vi "ROS_Status_Publisher_1.vi"() -> ()   [LabVIEW 2016]
uses:
  <userlib>/ROS for LabVIEW Software/ROS/Code/Console/Servers/ServerSubs/TopicDef.ctl
  <userlib>/ROS for LabVIEW Software/ROS/Code/SubVIs/_ROSDirection.ctl
  GlobalVI.vi
  <userlib>/ROS for LabVIEW Software/ROS/MessageBuilding/std_msgs/subs/stringScalar.vi
  <userlib>/ROS for LabVIEW Software/ROS/MessageBuilding/std_msgs/subs/float32Scalar.vi
  <userlib>/ROS for LabVIEW Software/ROS/MessageBuilding/std_msgs/subs/i32Scalar.vi
panel:
  out "JSON string 2":string
  out "error out":errorcluster
  out "UWB_error out":errorcluster
  out "JSON string":string
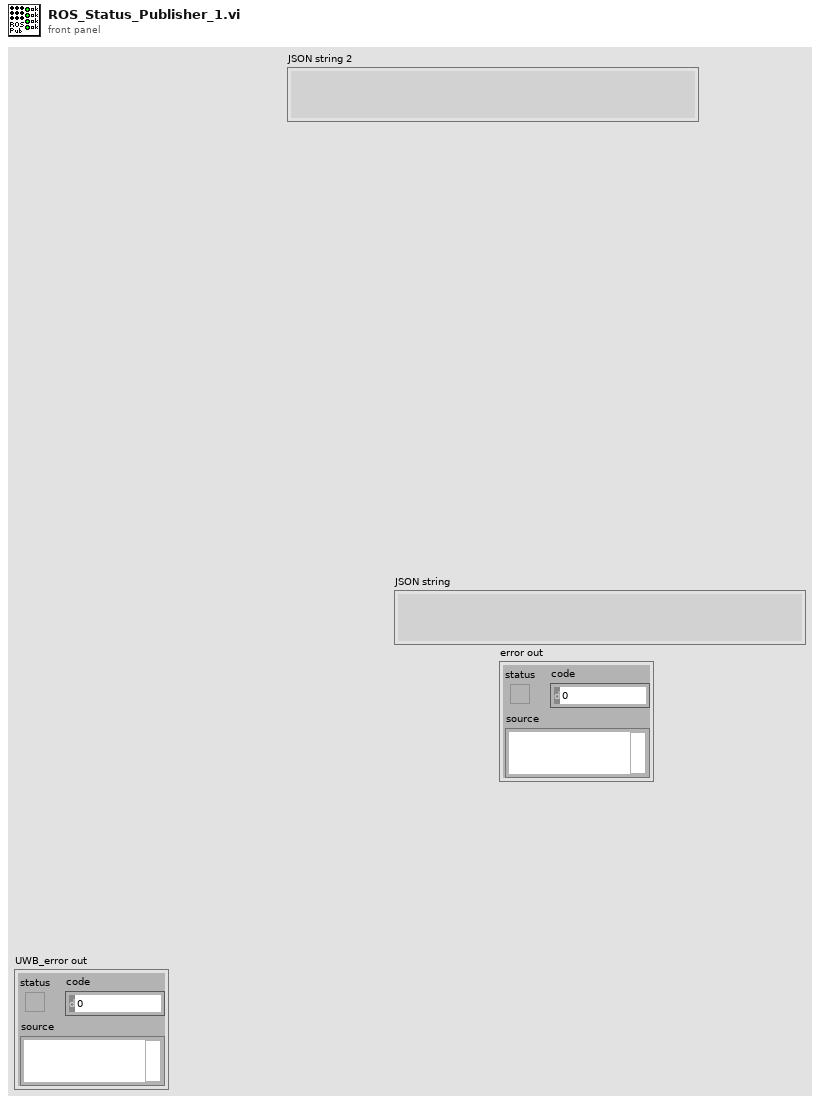
[diagram p1: front panel]
types:
  T1 = typedef "TopicDef.ctl" = cluster{"Topic":string, "Type":string, "Action":T2, "Update (ms)":u16, "queue size":u16}
  T2 = typedef "_ROSDirection.ctl" = enum16{"Node", "Publisher", "Subscriber", "ServiceClient", "ServiceProvider"}
  T3 = cluster{"status":cluster{"liftStatus":bool, "lidarBackStatus":bool, "uwbStatus":bool, "lightStatus":bool}}
  T4 = typedef "_ROSControl.ctl" = cluster{"topic port":u16, "Node":string, "topic":string, "type":string, "node port":u16, "error ":errorcluster, "Direction":T2, "Update (ms)":u16, "FIFO size":u16}
  T5 = cluster{"liftStatus":bool, "lidarBackStatus":bool, "uwbStatus":bool, "lightStatus":bool}
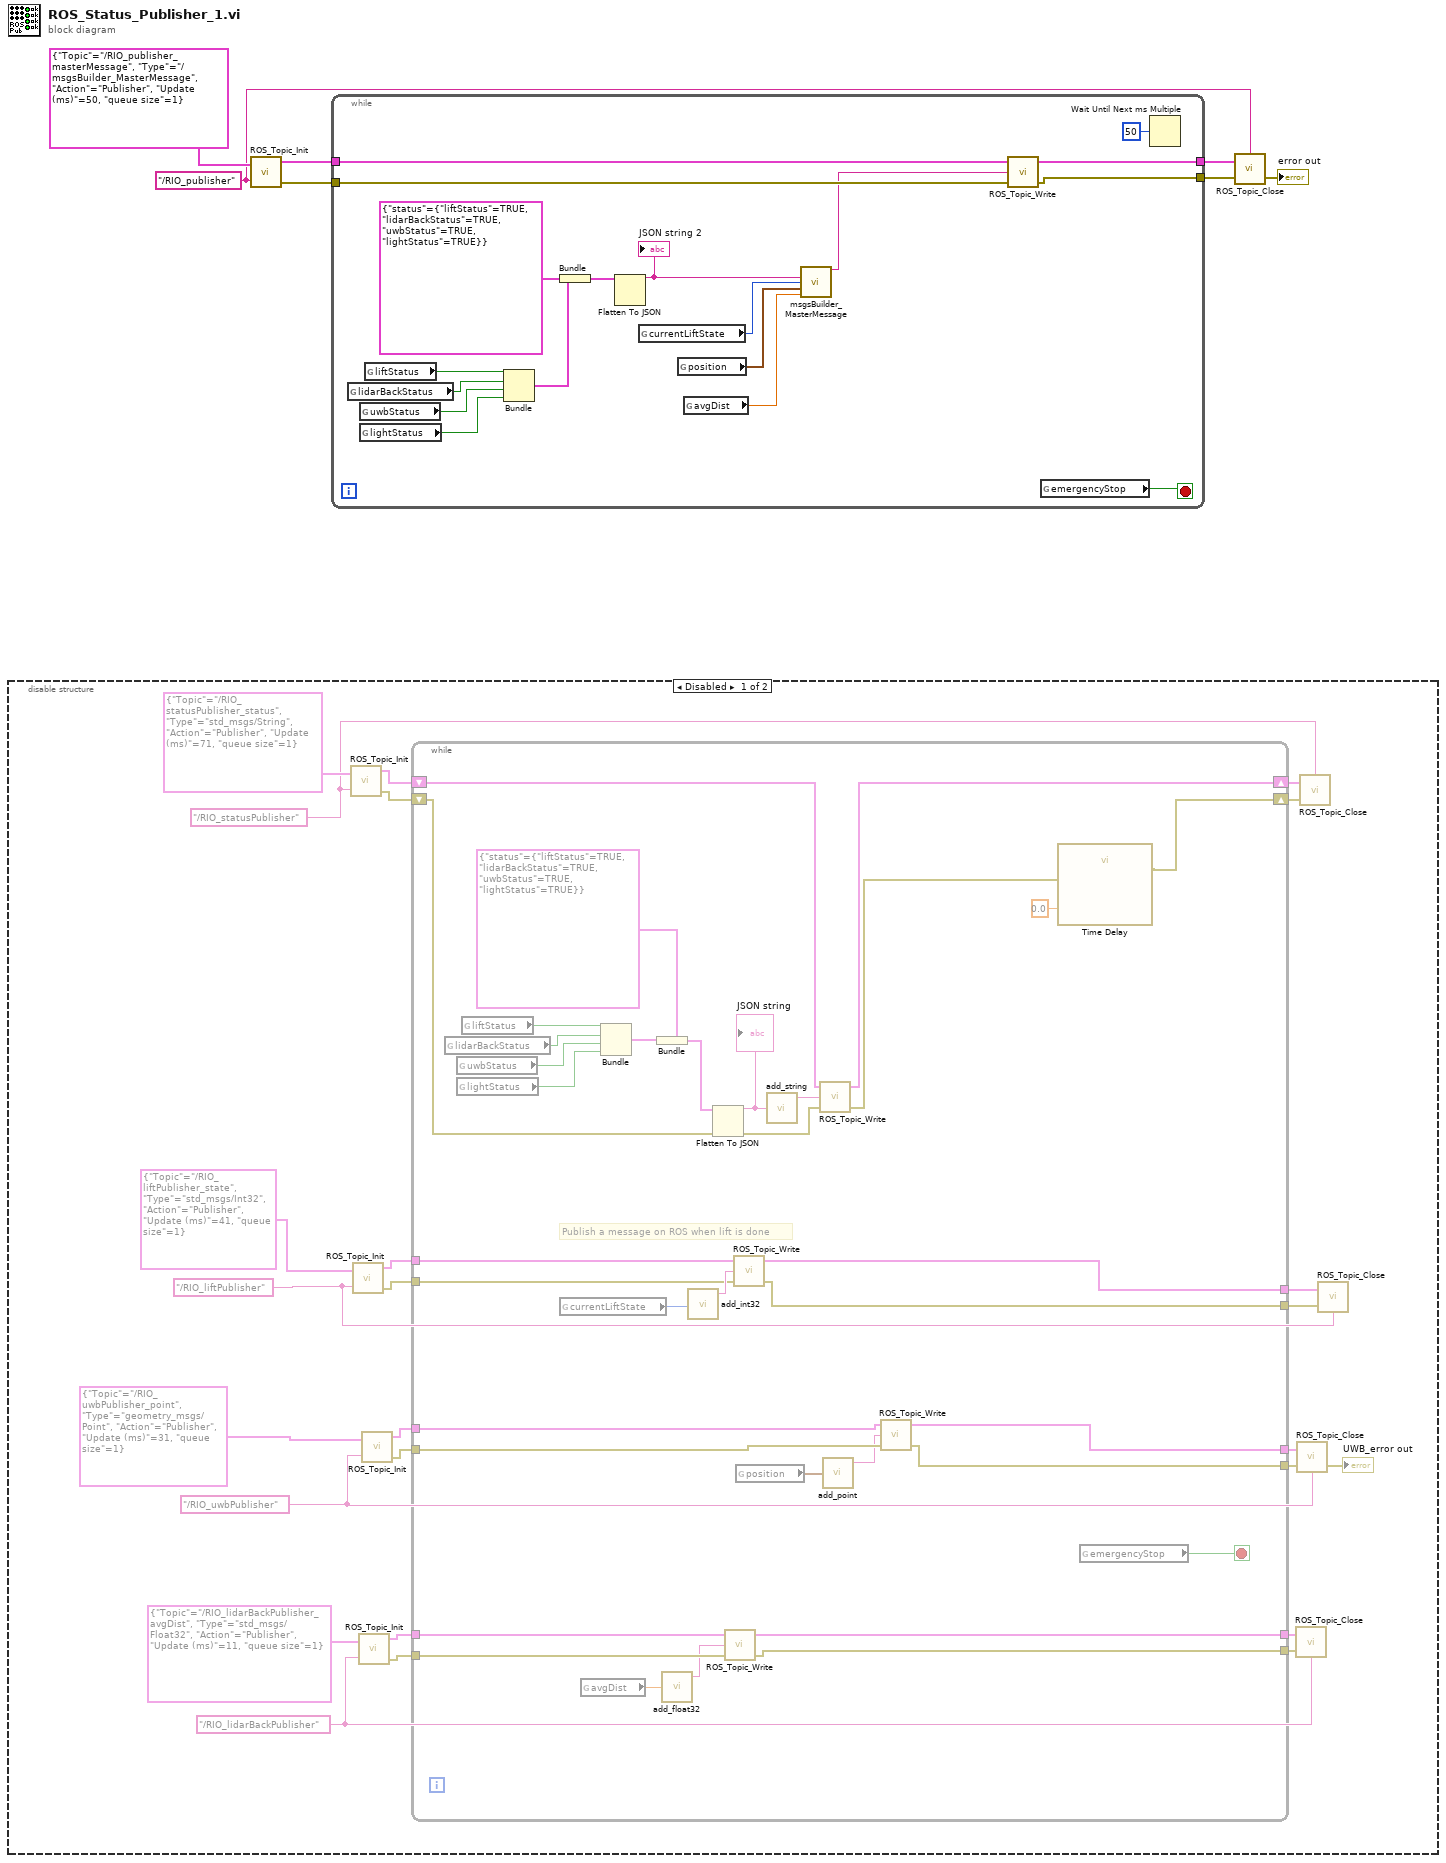
[diagram p0: block diagram]
diagram:
  w6 = "/RIO_publisher" ("node")
  n1 = disable-structure shown="Disabled" {
    frame Disabled {
      w12 = "/RIO_lidarBackPublisher" ("node")
      w14 = "/RIO_liftPublisher" ("node")
      w15 = "/RIO_uwbPublisher" ("node")
      w27 = "/RIO_statusPublisher" ("node")
      n2 = call <userlib>:"ROS_Topic_Init.vi"("Definitions"=T1 {"Topic"="/RIO_statusPublisher_status", "Type"="std_msgs/String", "Action"=enum."Publisher", "Update (ms)"=71, "queue size"=1}, "node"=w27) -> ("ROS out"=w31:T4, "error out"=w29:errorcluster)  [unwired: 1 in]
      n3 = call <userlib>:"ROS_Topic_Init.vi"("Definitions"=T1 {"Topic"="/RIO_liftPublisher_state", "Type"="std_msgs/Int32", "Action"=enum."Publisher", "Update (ms)"=41, "queue size"=1}, "node"=w14) -> ("ROS out"=w23:T4, "error out"=w22:errorcluster)  [unwired: 1 in]
      n4 = call <userlib>:"ROS_Topic_Init.vi"("Definitions"=T1 {"Topic"="/RIO_lidarBackPublisher_avgDist", "Type"="std_msgs/Float32", "Action"=enum."Publisher", "Update (ms)"=11, "queue size"=1}, "node"=w12) -> ("ROS out"=w10:T4, "error out"=w11:errorcluster)  [unwired: 1 in]
      n5 = call <userlib>:"ROS_Topic_Init.vi"("Definitions"=T1 {"Topic"="/RIO_uwbPublisher_point", "Type"="geometry_msgs/Point", "Action"=enum."Publisher", "Update (ms)"=31, "queue size"=1}, "node"=w15) -> ("ROS out"=w19:T4, "error out"=w18:errorcluster)  [unwired: 1 in]
      n6 = while {
        shift-right: [w66] -> w30
        shift-left: w31 -> [w67]
        shift-right: [w35] -> w28
        shift-left: w29 -> [w65]
        tunnel: w23 -> [w52]
        tunnel: w22 -> [w51]
        tunnel: [w50] -> w21
        tunnel: [w49] -> w20
        tunnel: w19 -> [w42]
        tunnel: w18 -> [w41]
        tunnel: [w40] -> w17
        tunnel: [w39] -> w16
        tunnel: w11 -> [w48]
        tunnel: w10 -> [w47]
        tunnel: [w46] -> w9
        tunnel: [w45] -> w8
        stop <- w36 stop-if-true
        # "Publish a message on ROS when lift is done"
        n7 = global read "GlobalVI.vi" "lidarBackStatus"() -> (w60:bool)
        n8 = global read "GlobalVI.vi" "uwbStatus"() -> (w59:bool)
        n9 = global read "GlobalVI.vi" "lightStatus"() -> (w58:bool)
        n10 = global read "GlobalVI.vi" "liftStatus"() -> (w61:bool)
        n11 = global read "GlobalVI.vi" "currentLiftState"() -> (w53:i32)
        n12 = global read "GlobalVI.vi" "avgDist"() -> (w43:sgl)
        n13 = Bundle("liftStatus"=w61, "lidarBackStatus"=w60, "uwbStatus"=w59, "lightStatus"=w58) -> (w57:T5)  [unwired: 1 in]
        n14 = Bundle(cluster=T3 {"status"={"liftStatus"=TRUE, "lidarBackStatus"=TRUE, "uwbStatus"=TRUE, "lightStatus"=TRUE}}, "status"=w57) -> (w56:T3)
        n15 = call-poly <userlib>:"add_float32.vi"("Numeric"=w43) -> ("msg out"=w44:string)  [unwired: 4 in]
        n16 = call-poly <userlib>:"add_int32.vi"("Numeric"=w53) -> ("msg out"=w54:string)  [unwired: 4 in]
        n17 = Flatten To JSON(anything=w56, error in (no error)=w65) -> (JSON string=w63:string, 11:w62:errorcluster)  [unwired: 1 in]
        "JSON string" <- w63
        n18 = call <userlib>:"ROS_Topic_Write.vi"("error in (no error)"=w48, "Msg in"=w44, "ROS in"=w47) -> ("error out"=w45:errorcluster, "ROS out"=w46:T4)  [unwired: 1 in]
        n19 = call <userlib>:"ROS_Topic_Write.vi"("error in (no error)"=w51, "Msg in"=w54, "ROS in"=w52) -> ("error out"=w50:errorcluster, "ROS out"=w49:T4)  [unwired: 1 in]
        n20 = global read "GlobalVI.vi" "position"() -> (w38:cluster{"x":dbl, "y":dbl, "z":dbl})
        n21 = call-poly <userlib>:"add_string.vi"("String"=w63) -> ("msg out"=w64:string)  [unwired: 4 in]
        n22 = call <userlib>:"ROS_Topic_Write.vi"("error in (no error)"=w62, "Msg in"=w64, "ROS in"=w67) -> ("error out"=w34:errorcluster, "ROS out"=w66:T4)  [unwired: 1 in]
        n23 = call <userlib>:"add_point.vi"("Point"=w38) -> ("msg out"=w37:string)  [unwired: 4 in]
        n24 = call <userlib>:"ROS_Topic_Write.vi"("error in (no error)"=w41, "Msg in"=w37, "ROS in"=w42) -> ("error out"=w40:errorcluster, "ROS out"=w39:T4)  [unwired: 1 in]
        n25 = call "Time Delay"("error in (no error)"=w34, "Delay Time (s)"=0.0) -> ("error out"=w35:errorcluster)  [unwired: 9 in]
        n26 = global read "GlobalVI.vi" "emergencyStop"() -> (w36:bool)
      }
      n27 = call <userlib>:"ROS_Topic_Close.vi"("error in"=w8, "ROS in"=w9, "node"=w12) -> ()  [unwired: 1 in, 1 out]
      n28 = call <userlib>:"ROS_Topic_Close.vi"("error in"=w17, "ROS in"=w16, "node"=w15) -> ("error out"=→"UWB_error out":errorcluster)  [unwired: 1 in]
      n29 = call <userlib>:"ROS_Topic_Close.vi"("error in"=w28, "ROS in"=w30, "node"=w27) -> ()  [unwired: 1 in, 1 out]
      n30 = call <userlib>:"ROS_Topic_Close.vi"("error in"=w21, "ROS in"=w20, "node"=w14) -> ()  [unwired: 1 in, 1 out]
    }
    frame Enabled {
    }
  }
  n31 = call <userlib>:"ROS_Topic_Init.vi"("Definitions"=T1 {"Topic"="/RIO_publisher_masterMessage", "Type"="/msgsBuilder_MasterMessage", "Action"=enum."Publisher", "Update (ms)"=50, "queue size"=1}, "node"=w6) -> ("ROS out"=w5:T4, "error out"=w3:errorcluster)  [unwired: 1 in]
  n32 = while {
    tunnel: w5 -> [w85]
    tunnel: [w84] -> w4
    tunnel: w3 -> [w83]
    tunnel: [w82] -> w2
    stop <- w69 stop-if-true
    n33 = global read "GlobalVI.vi" "lidarBackStatus"() -> (w76:bool)
    n34 = global read "GlobalVI.vi" "uwbStatus"() -> (w77:bool)
    n35 = global read "GlobalVI.vi" "lightStatus"() -> (w78:bool)
    n36 = global read "GlobalVI.vi" "liftStatus"() -> (w75:bool)
    n37 = Bundle("liftStatus"=w75, "lidarBackStatus"=w76, "uwbStatus"=w77, "lightStatus"=w78) -> (w79:T5)  [unwired: 1 in]
    n38 = Bundle(cluster=T3 {"status"={"liftStatus"=TRUE, "lidarBackStatus"=TRUE, "uwbStatus"=TRUE, "lightStatus"=TRUE}}, "status"=w79) -> (w80:T3)
    n39 = Flatten To JSON(anything=w80) -> (JSON string=w74:string)  [unwired: 2 in, 1 out]
    "JSON string 2" <- w74
    n40 = global read "GlobalVI.vi" "currentLiftState"() -> (w73:i32)
    n41 = global read "GlobalVI.vi" "position"() -> (w72:cluster{"x":dbl, "y":dbl, "z":dbl})
    n42 = global read "GlobalVI.vi" "avgDist"() -> (w71:sgl)
    n43 = call "msgsBuilder_MasterMessage.vi"("statusString"=w74, "liftState"=w73, "position"=w72, "avgDist"=w71) -> ("msg out"=w70:string)  [unwired: 11 in]
    n44 = call <userlib>:"ROS_Topic_Write.vi"("error in (no error)"=w83, "Msg in"=w70, "ROS in"=w85) -> ("error out"=w82:errorcluster, "ROS out"=w84:T4)  [unwired: 1 in]
    n45 = global read "GlobalVI.vi" "emergencyStop"() -> (w69:bool)
    n46 = Wait Until Next ms Multiple(millisecond multiple=u32 50) -> ()  [unwired: 1 out]
  }
  n47 = call <userlib>:"ROS_Topic_Close.vi"("error in"=w2, "ROS in"=w4, "node"=w6) -> ("error out"=→"error out":errorcluster)  [unwired: 1 in]
